vi "ParseUserFunctions.vi"(8 "error in (no error)":errorcluster, 10 "User defined functions in":string, 11 "FunctionMenu in":refnum<class "InsertFunctionMenu.lvclass">) -> (0 "error out":errorcluster, 3 "FunctionMenu out":refnum<class "InsertFunctionMenu.lvclass">)   [LabVIEW 2013, in "InsertFunctionMenu.lvclass"]
uses:
  InsertFunctionMenu.lvclass
  InsertFunctionMenu.lvclass/InsertFunctionMenu.ctl
  <vilib>/regexp/Match Regular Expression.xnode
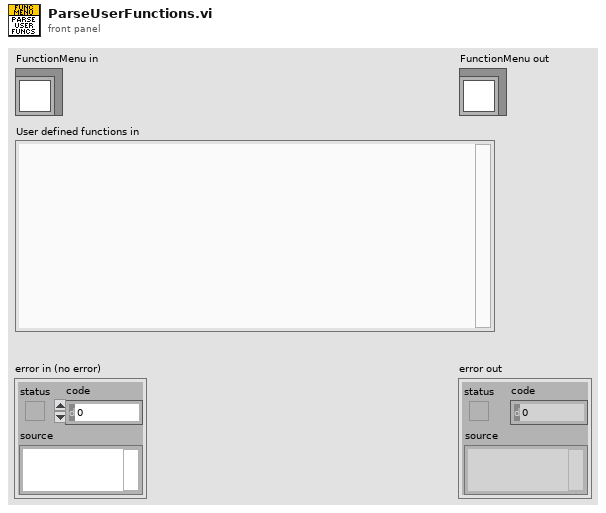
[diagram p1: front panel]
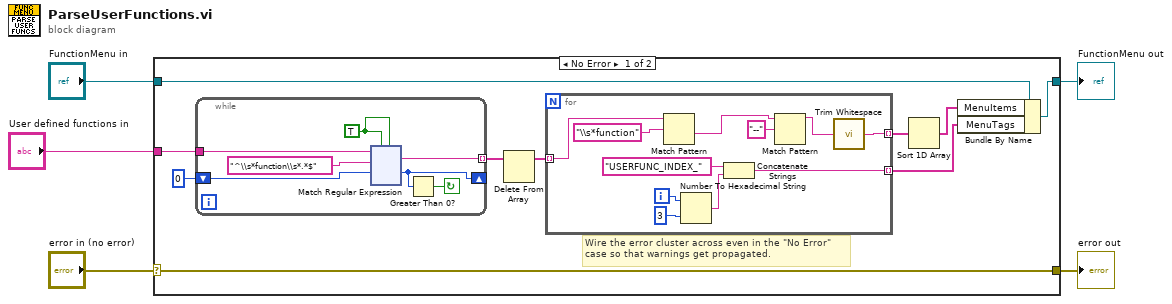
[diagram p0: block diagram]
diagram:
  n1 = case shown="No Error" "error in (no error)" {
    selector: "error in (no error)" -> [w15 w149]
    tunnel: [w15 w149] -> w4
    tunnel: [w8 w148] -> w2
    tunnel: "FunctionMenu in" -> [w9 w148]
    tunnel: "User defined functions in" -> [w10 _]
    frame No Error {
      # "Wire the error cluster across even in the \"No Error\"\ncase so that warnings get propagated."
      n2 = while {
        tunnel: [w32] -> w13 mode=indexing
        tunnel: w10 -> [w31]
        shift-right: [w29] -> _
        shift-left: 0 ("offset past match") -> [w30]
        stop <- w33 continue-if-true
        w27 = TRUE ("ignore case? (F)")
        n3 = xnode "Match Regular Expression"("input string"=w31, "regular expression"="^\\s*function\\s*.*$", "offset (0)"=w30, "ignore case? (F)"=w27, "multiline? (F)"=w27) -> ("whole match"=w32:string, "offset past match"=w29:i32)  [unwired: 1 in, 3 out]
        n4 = Greater Than 0?(x=w29) -> (x > 0?=w33:bool)
      }
      n5 = Delete From Array(array=w13) -> (array with subset deleted=w12:string[])  [unwired: 2 in, 1 out]
      n6 = for {
        tunnel: [w22] -> w11 mode=indexing
        tunnel: w12 -> [w25] mode=indexing
        tunnel: [w19] -> w6 mode=indexing
        i -> [w24]
        n7 = Match Pattern(string=w25, regular expression="\\s*function") -> (after substring=w17:string)  [unwired: 1 in, 3 out]
        n8 = Number To Hexadecimal String(1:u32 3 ("default (0 U32)"), 2:w24) -> (0:w20:string)
        n9 = Concatenate Strings("USERFUNC_INDEX_" ("string"), w20) -> (w19:string)
        n10 = Match Pattern(string=w17, regular expression="--") -> (before substring=w16:string)  [unwired: 1 in, 3 out]
        n11 = call <vilib>:"Trim Whitespace.vi"("string"=w16) -> ("trimmed string"=w22:string)  [unwired: 1 in]
      }
      n12 = Sort 1D Array(array=w11) -> (sorted array=w7:string[])
      n13 = Bundle By Name(cluster=w9, "MenuItems"=w7, "MenuTags"=w6) -> (w8:refnum<class "InsertFunctionMenu.lvclass">)
    }
    frame Error {
    }
  }
  "error out" <- w4
  "FunctionMenu out" <- w2
